vi "GoTo.vi"(8 "error in":errorcluster, 11 "control refs":T1) -> (0 "error out":errorcluster, 2 "VisibleValue":u64)   [LabVIEW 2017]
panel:
  in  "Go":bool
  in  "Index":u64 max=998
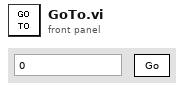
[diagram p1: front panel]
types:
  T1 = cluster{"Tree":refnum<vi>, "Tab Control":refnum<vi>, "property list":refnum<vi>, "raw data list":refnum<vi>, "Waveform Graph":refnum<vi>, "Ok":refnum<vi>, "Ok 2":refnum<vi>, "Ok 3":refnum<vi>, "Ok 4":refnum<vi>, "Scrollbar":refnum<vi>, "Ok 5":refnum<vi>, "TopLeftValue":refnum<vi>, "TotalCount":refnum<vi>}
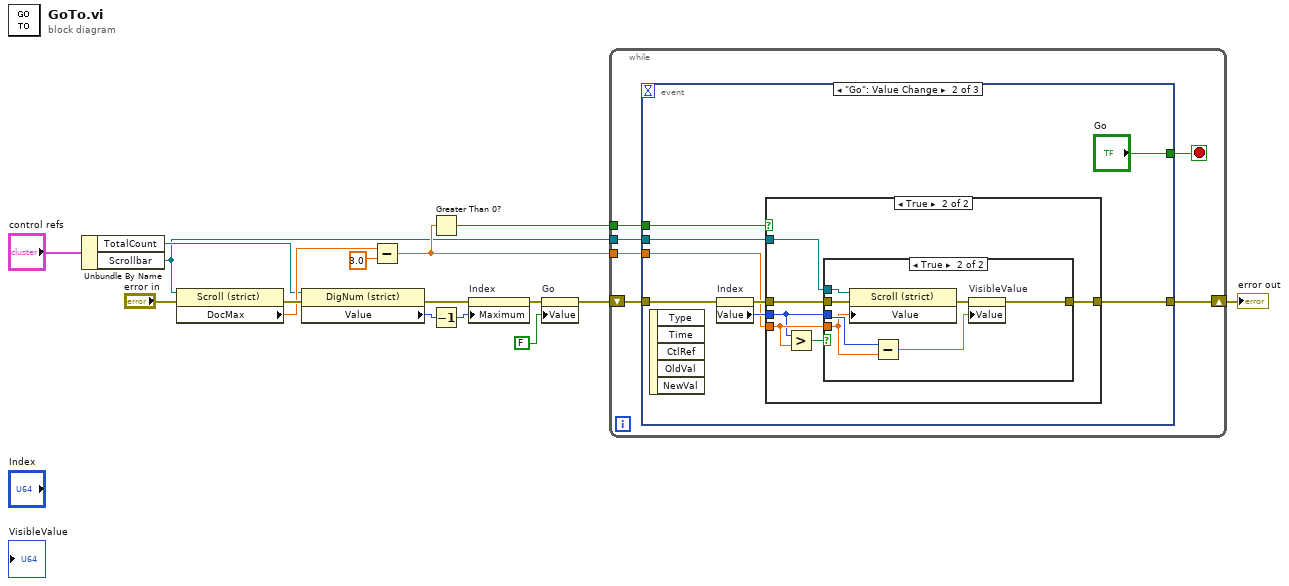
[diagram p0: block diagram]
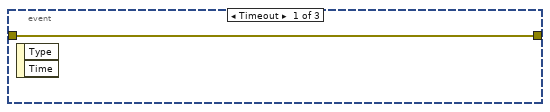
[diagram p2: hidden frame]
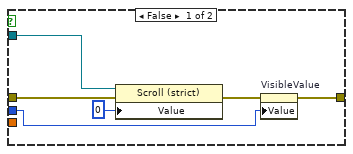
[diagram p3: hidden frame]
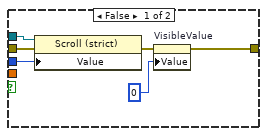
[diagram p4: hidden frame]
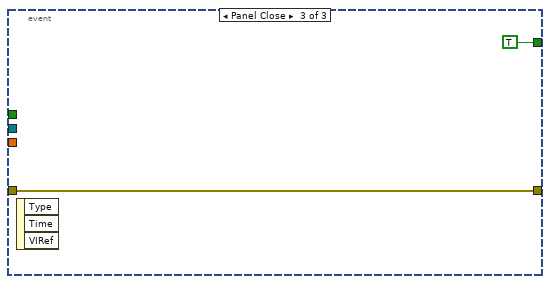
[diagram p5: hidden frame]
diagram:
  n1 = Unbundle By Name("control refs") -> ("TotalCount"=w7:refnum<vi>, "Scrollbar"=w5:refnum<vi>)
  n2 = property on="Property Node" class="Scroll (strict)"(reference=w5, error in="error in") -> (error out=w13:errorcluster, "DocMax"=w12:dbl)  [unwired: 1 out]
  n3 = property on="Property Node" class="DigNum (strict)"(reference=w7, error in=w13) -> (error out=w2:errorcluster, "Value"=w1:u64)  [unwired: 1 out]
  n4 = Subtract(x=w12, y=3.0) -> (x-y=w6:dbl)
  n5 = Greater Than 0?(x=w6) -> (x > 0?=w8:bool)
  n6 = Decrement(x=w1) -> (x-1=w3:u64)
  n7 = property on="Index" class="DigNum (strict)"(error in=w2, "Maximum"=w3) -> (error out=w9:errorcluster)  [unwired: 1 in, 1 out]
  n8 = property on="Go" class="Bool (strict)"(error in=w9, "Value"=FALSE ("Visible")) -> (error out=w15:errorcluster)  [unwired: 1 in, 1 out]
  n9 = while {
    shift-right: [w20] -> w14
    shift-left: w15 -> [w21]
    tunnel: w8 -> [w19]
    tunnel: w6 -> [w18]
    tunnel: w5 -> [w17]
    stop <- w22 stop-if-true
    n10 = event shown="[1] \"Go\": Value Change" {
      selector: _ -> [_ _ _]
      dyn-events: _ -> [_ _ _]
      timeout: _ -> [_ _ _]
      tunnel: [_ "Go" TRUE ("OK Button")] -> w22
      tunnel: w21 -> [w23 w31 w57]
      tunnel: [w23 w26 w57] -> w20
      tunnel: w19 -> [_ w29 _]
      tunnel: w18 -> [_ w25 _]
      tunnel: w17 -> [_ w24 _]
      event Timeout {
        n11 = event-data() -> ()  [unwired: 1 in, 2 out]
      }
      event "Go": Value Change {
        n12 = event-data() -> ()  [unwired: 1 in, 5 out]
        n13 = property on="Index" class="DigNum (strict)"(error in=w31) -> (error out=w28:errorcluster, "Value"=w27:u64)  [unwired: 1 in, 1 out]
        n14 = case shown="True" w29 {
          tunnel: w28 -> [w36 w40]
          tunnel: w27 -> [w32 w41]
          tunnel: [w37 w39] -> w26
          tunnel: w25 -> [_ w42]
          tunnel: w24 -> [w33 w38]
          frame False {
            n15 = property on="Property Node" class="Scroll (strict)"(reference=w33, error in=w36, "Value"=u64 0 ("ScrollBarIndex")) -> (error out=w35:errorcluster)  [unwired: 1 out]
            n16 = property on="VisibleValue" class="DigNum (strict)"(error in=w35, "Value"=w32) -> (error out=w37:errorcluster)  [unwired: 1 in, 1 out]
          }
          frame True {
            n17 = Greater?(x=w41, y=w42) -> (0:w43:bool)
            n18 = case shown="True" w43 {
              tunnel: w42 -> [_ w50]
              tunnel: w41 -> [w44 w56]
              tunnel: w40 -> [w46 w52]
              tunnel: [w48 w54] -> w39
              tunnel: w38 -> [w45 w51]
              frame False {
                n19 = property on="Property Node" class="Scroll (strict)"(reference=w45, error in=w46, "Value"=w44) -> (error out=w47:errorcluster)  [unwired: 1 out]
                n20 = property on="VisibleValue" class="DigNum (strict)"(error in=w47, "Value"=u64 0 ("VisibleValue")) -> (error out=w48:errorcluster)  [unwired: 1 in, 1 out]
              }
              frame True {
                n21 = property on="Property Node" class="Scroll (strict)"(reference=w51, error in=w52, "Value"=w50) -> (error out=w53:errorcluster)  [unwired: 1 out]
                n22 = Subtract(x=w56, y=w50) -> (x-y=w55:dbl)
                n23 = property on="VisibleValue" class="DigNum (strict)"(error in=w53, "Value"=w55) -> (error out=w54:errorcluster)  [unwired: 1 in, 1 out]
              }
            }
          }
        }
      }
      event Panel Close {
        n24 = event-data() -> ()  [unwired: 1 in, 3 out]
      }
    }
  }
  "error out" <- w14
